vi "rmp_main.vi"(6 "rmp.p.simIn":T2 {"rmp.p.procVar" format="%#_13g"}, 7 "rmp.i.externalTrigger":bool, 8 "rmp.p.reset":T1, 9 "rmp.p.action":cluster{"rmp.p.start":bool, "rmp.p.stop":bool}, 10 "rmp.p.triggerParams":T5 {"rmp.triggerSource" items=["Absolute z height", "Process variable", "External"]}, 11 "rmp.p.params":T4) -> (0 "rmp.s.running":bool, 3 "rmp.o.height":T3)   [LabVIEW 2016]
uses:
  <vilib>/rvi/Emulation/niFpgaEmulationIsFPGAContextNoSignature.vi
  <vilib>/rvi/Emulation/niFpgaSctlEmulationGetInTimedLoop.vi
  <vilib>/rvi/errors/niFpgaSetErrorForExecOnDevCompSimple.vi
  <vilib>/rvi/eio/common/nirviEmuReportErrorAndStop.vi
  <vilib>/rvi/DataTransferAndStorage/Container/Common/niFpgaContainerGetUniqueNameForEmu.vi
  <vilib>/rvi/FIFO/Fifo_Resource/nirvififoEmulationSetSize.vi
  <vilib>/rvi/FIFO/Fifo_Resource/nirviFifoEmulationQueueMgr.vi
  <instcachedir>/0/nirviFifoEmulationQueueMgr_E5CAEC123FF24DC58D834DCA3CDAA9B5.lvgen/nirviFifoEmulationQueueMgr_E5CAEC123FF24DC58D834DCA3CDAA9B5_009.vi
  <vilib>/rvi/FIFO/Fifo_Resource/nirvififoEmulationDetermineInputValidOut.vi
  <vilib>/rvi/FIFO/Fifo_Resource/nirvififoEmulationCreateLock.vi
  <vilib>/rvi/Emulation/niFpgaProcessEmulError.vi
  <vilib>/rvi/FIFO/Fifo_Resource/nirvififoEmulationObtainLock.vi
  <vilib>/rvi/FIFO/Fifo_Resource/nirvififoEmulationReleaseLock.vi
  <vilib>/rvi/occurrence/nirviWaitOnOccurrenceBase.vi
  <vilib>/rvi/errors/nirviReportUnexpectedCaseInternalError.vi
  <vilib>/rvi/errors/nirviReportUnexpectedCaseInternalError (U32).vi
  <vilib>/rvi/Memory/Memory_Emulation/niFpgaMemoryEmulationCacheClearOnFirstRun.vi
  <vilib>/rvi/Memory/Memory_Emulation/nirvimemoryEmulationManagerCache_MakeExclusive.vi
  <vilib>/rvi/Memory/Memory_Emulation/niFpgaMemoryEmulationValidateCache.vi
  <vilib>/rvi/Memory/Memory_Emulation/nirvimemoryEmulationManagerCache_InsertValue.vi
  <vilib>/Utility/error.llb/Clear Errors.vi
  <vilib>/rvi/Memory/Memory_Emulation/nirvimemoryEmulationManagerCache_ReleaseExclusive.vi
  <vilib>/rvi/Memory/Memory_Emulation/nirvimemoryEmulationManagerCache_GetValue.vi
  <vilib>/rvi/Memory/Memory_Emulation/nirvimemoryEmulationManagerCache_SetValue.vi
  <instcachedir>/0/nirviFifoEmulationQueueMgr_E5CAEC123FF24DC58D834DCA3CDAA9B5.lvgen/nirviFifoEmulationQueueMgr_E5CAEC123FF24DC58D834DCA3CDAA9B5_000.vi
  <vilib>/rvi/DataTransferAndStorage/Container/XNode/niFpgaContainer.xnode
  <vilib>/rvi/FIFO/Fifo_Resource/nirvififoEmulationWrite.vi
  <vilib>/rvi/DataTransferAndStorage/Register/Emulation/niFpgaRegisterEmulation.vi
  <vilib>/rvi/FIFO/Fifo_Resource/nirvififoEmulationRead.vi
  <vilib>/rvi/FXPMathLib/FxpAdd/XNode/nifxpmath_Add.xnode
  <instrlib>/_niInstr/Basic Elements/v1/FPGA/niInstr Basic Elements v1 FPGA.lvlib
  <vilib>/rvi/FXPMathLib/sim/FxpSim.dll
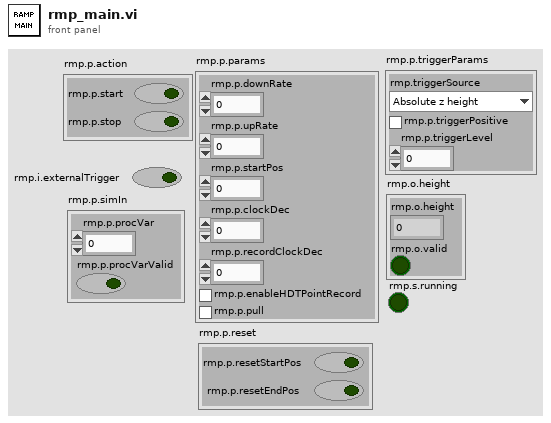
[diagram p1: front panel]
types:
  T1 = cluster{"rmp.p.resetStartPos":bool, "rmp.p.resetEndPos":bool}
  T2 = cluster{"rmp.p.procVar":fxp<+/-,24,16>, "rmp.p.procVarValid":bool}
  T3 = cluster{"rmp.o.height":fxp<+/-,24,2>, "rmp.o.valid":bool}
  T4 = cluster{"rmp.p.downRate":fxp<+/-,22,-10>, "rmp.p.upRate":fxp<+/-,22,-10>, "rmp.p.startPos":fxp<+/-,24,2>, "rmp.p.clockDec":u16, "rmp.p.recordClockDec":u16, "rmp.p.enableHDTPointRecord":bool, "rmp.p.pull":bool}
  T5 = cluster{"rmp.triggerSource":u8, "rmp.p.triggerPositive":bool, "rmp.p.triggerLevel":fxp<+/-,24,16>}
  T6 = cluster{"x+y":fxp<+/-,35,3>, "output valid":bool}
  T7 = cluster{"Element":fxp<+/-,24,16>, "Output Valid":bool}
  T8 = cluster{"rmp.p.triggerLevel":fxp<+/-,24,16>, "rmp.i.externalTrigger":bool}
  T9 = cluster{"Element":fxp<+/-,48,16>, "rmp.i.externalTrigger":bool}[]
  T10 = cluster{"Element":fxp<+/-,48,16>, "rmp.i.externalTrigger":bool}
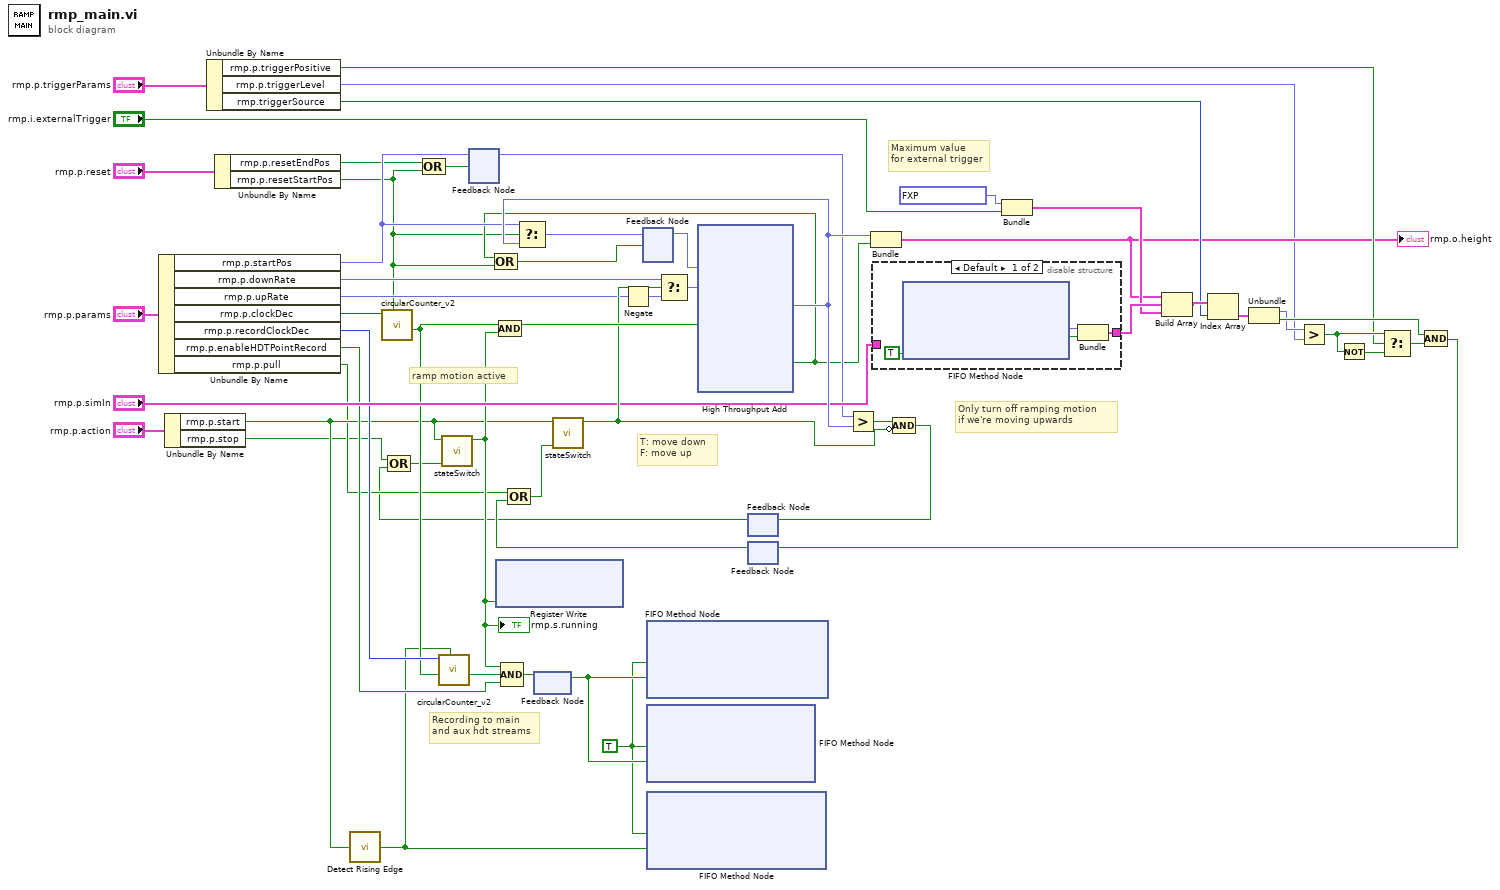
[diagram p0: block diagram]
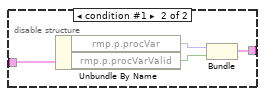
[diagram p2: hidden frame]
diagram:
  w1 = TRUE ("Element")
  # "Recording to main\nand aux hdt streams"
  # "Maximum value \nfor external trigger"
  # "Only turn off ramping motion\nif we're moving upwards"
  # "T: move down\nF: move up"
  # "ramp motion active"
  n1 = Unbundle By Name("rmp.p.params") -> ("rmp.p.startPos"=w19:fxp<+/-,24,2>, "rmp.p.downRate"=w20:fxp<+/-,22,-10>, "rmp.p.upRate"=w30:fxp<+/-,22,-10>, "rmp.p.clockDec"=w29:u16, "rmp.p.recordClockDec"=w26:u16, "rmp.p.enableHDTPointRecord"=w22:bool, "rmp.p.pull"=w11:bool)
  n2 = Unbundle By Name("rmp.p.action") -> ("rmp.p.start"=w13:bool, "rmp.p.stop"=w8:bool)
  n3 = Unbundle By Name("rmp.p.triggerParams") -> ("rmp.p.triggerPositive"=w32:bool, "rmp.p.triggerLevel"=w21:fxp<+/-,24,16>, "rmp.triggerSource"=w33:u8)
  n4 = Unbundle By Name("rmp.p.reset") -> ("rmp.p.resetEndPos"=w5:bool, "rmp.p.resetStartPos"=w4:bool)
  n5 = call <instrlib>:"Detect Rising Edge.vi"("signal"=w13) -> ("edge detected"=w3:bool)  [unwired: 14 in]
  n6 = call "circularCounter_v2.vi"("reset"=w4, "maxCount"=w29) -> ("maxPulse"=w25:bool)  [unwired: 6 in, 3 out]
  n7 = Compound Arithmetic op=OR(w5, w4) -> (w7:bool)
  n8 = call "circularCounter_v2.vi"("reset"=w3, "doStep"=w25, "maxCount"=w26) -> ("maxPulse"=w24:bool)  [unwired: 5 in, 3 out]
  n9 = feedback #1() -> (w18:fxp<+/-,24,2>)  [unwired: 1 in]
  n10 = feedback-in #1(w19, w7) -> ()
  n11 = feedback #2() -> (w2:bool)  [unwired: 1 in]
  n12 = Negate(x=w30) -> (-x=w56:fxp<+/-,23,-9>)
  n13 = feedback #3() -> (w55:fxp<+/-,35,3>)  [unwired: 1 in]
  n14 = xnode ("FIFO Method Node")("Element"=w1, "Input Valid"=w2) -> ()  [unwired: 1 in, 2 out]
  n15 = xnode ("FIFO Method Node")("Element"=w1, "Input Valid"=w2) -> ()  [unwired: 1 in, 2 out]
  n16 = xnode ("FIFO Method Node")("Element"=w1, "Input Valid"=w3) -> ()  [unwired: 1 in, 2 out]
  n17 = feedback #4() -> (w9:bool)  [unwired: 1 in]
  n18 = Compound Arithmetic op=OR(w8, w9) -> (w16:bool)
  n19 = call "stateSwitch.vi"("disable"=w16, "enable"=w13) -> ("state"=w14:bool)  [unwired: 9 in]
  "rmp.s.running" <- w14
  n20 = xnode ("Register Write")("Data"=w14) -> ()  [unwired: 1 in, 1 out]
  n21 = Compound Arithmetic op=AND(w25, w14) -> (w49:bool)
  n22 = Compound Arithmetic op=AND(w14, w24, w22) -> (w23:bool)
  n23 = feedback-in #2(w23) -> ()
  n24 = feedback #5() -> (w12:bool)  [unwired: 1 in]
  n25 = Compound Arithmetic op=OR(w11, w12) -> (w10:bool)
  n26 = call "stateSwitch.vi"("disable"=w10, "enable"=w13) -> ("state"=w46:bool)  [unwired: 9 in]
  n27 = Select(t=w20, s=w46, f=w56) -> (s? t:f=w54:fxp<+/-,23,-9>)
  n28 = xnode ("High Throughput Add")("x"=w55, "y"=w54, "input valid"=w49) -> ("x+y"=w42:fxp<+/-,35,3>, "output valid"=w17:bool)  [unwired: 1 in, 1 out]
  n29 = Compound Arithmetic op=OR(w17, w4) -> (w52:bool)
  n30 = Select(t=w19, s=w4, f=w42) -> (s? t:f=w53:fxp<+/-,35,3>)
  n31 = feedback-in #3(w53, w52) -> ()
  n32 = Greater?(x=w18, y=w42) -> (0:w48:bool)
  n33 = Bundle("x+y"=w42, "output valid"=w17) -> (w27:T6)  [unwired: 1 in]
  "rmp.o.height" <- w27
  n34 = disable-structure shown="Default" {
    disable-tunnel: [w58 w64] -> w44
    disable-tunnel: "rmp.p.simIn" -> [_ w63]
    frame condition #0 (active) {
      n35 = xnode ("FIFO Method Node")("Ready for Output"=TRUE) -> ("Element"=w60:fxp<+/-,24,16>, "Output Valid"=w59:bool)  [unwired: 1 in, 1 out]
      n36 = Bundle("Element"=w60, "Output Valid"=w59) -> (w58:T7)  [unwired: 1 in]
    }
    frame condition #1 {
      n37 = Unbundle By Name(w63) -> ("rmp.p.procVar"=w62:fxp<+/-,24,16>, "rmp.p.procVarValid"=w61:bool)
      n38 = Bundle("rmp.p.procVar"=w62, "rmp.p.procVarValid"=w61) -> (w64:T2)  [unwired: 1 in]
    }
  }
  n39 = Compound Arithmetic op=AND(w48, invert w46) -> (w47:bool)
  n40 = feedback-in #4(w47) -> ()
  n41 = Bundle("rmp.p.triggerLevel"=fxp<+/-,24,16> 32767.99609375, "rmp.i.externalTrigger"="rmp.i.externalTrigger") -> (w37:T8)  [unwired: 1 in]
  n42 = Build Array(w27, w44, w37) -> (w43:T9)
  n43 = Index Array(array=w43, index=w33) -> (element=w39:T10)
  n44 = Unbundle(w39) -> ("Element"=w38:fxp<+/-,48,16>, "rmp.i.externalTrigger"=w40:bool)
  n45 = Greater?(x=w38, y=w21) -> (0:w50:bool)
  n46 = Not(x=w50) -> (.not. x?=w51:bool)
  n47 = Select(t=w50, s=w32, f=w51) -> (s? t:f=w45:bool)
  n48 = Compound Arithmetic op=AND(w40, w45) -> (w41:bool)
  n49 = feedback-in #5(w41) -> ()
